vi "3-Random number on meter.vi"() -> ()   [LabVIEW 2019]
panel:
  in  "Sampling time in ms":u32=1000
  out "?":dbl(knob)=0.28909456036973413 scale=0.0..1.0
  in  "?":bool
  # "RANDOM NUMBER GENERATOR"
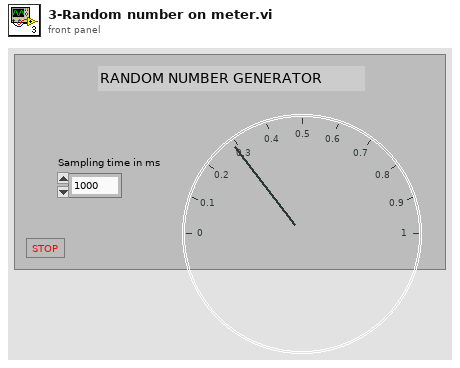
[diagram p1: front panel]
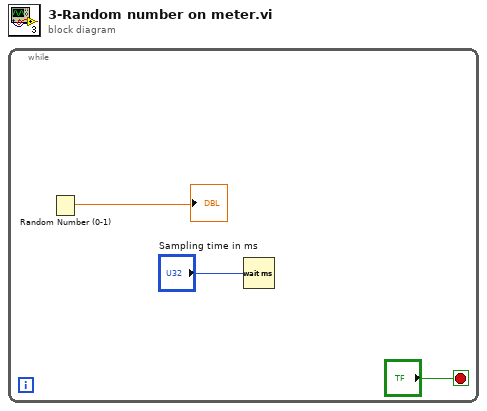
[diagram p0: block diagram]
diagram:
  n1 = while {
    stop <- "?" stop-if-true
    n2 = Random Number (0-1)() -> (number: 0 to 1=→"?":dbl)
    n3 = Wait (ms)(milliseconds to wait="Sampling time in ms") -> ()  [unwired: 1 out]
  }
